vi "Problem 10.vi"() -> ()   [LabVIEW 2013, in "Problem 10.lvlib"]
uses:
  Problem 10.lvlib
  Problem 3/Problem 3.lvlib
panel:
  out "Sum of Primes <2M":u64
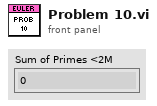
[diagram p1: front panel]
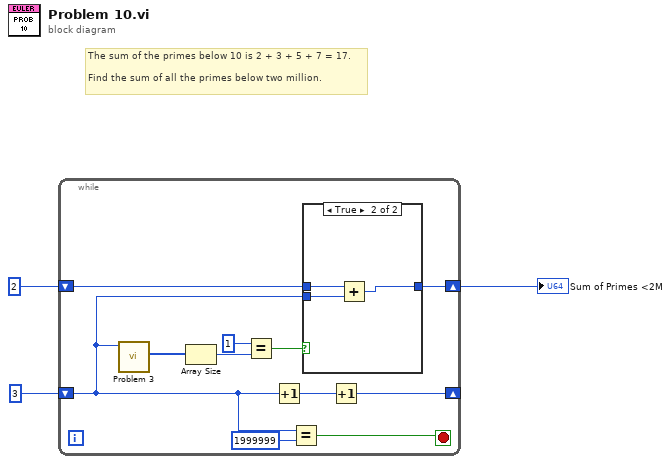
[diagram p0: block diagram]
diagram:
  # "The sum of the primes below 10 is 2 + 3 + 5 + 7 = 17.\n\nFind the sum of all the primes below two million."
  n1 = while {
    shift-right: [w7] -> _
    shift-left: u64 3 -> [w6]
    shift-right: [w9] -> w1
    shift-left: u64 2 -> [w11]
    stop <- w4 stop-if-true
    n2 = call "Problem 3.vi"("Number to Factor"=w6) -> ("List of Factors"=w14:u64[])  [unwired: 9 in, 1 out]
    n3 = Array Size(array=w14) -> (size(s)=w13:i32)
    n4 = Equal?(x=1, y=w13) -> (x = y?=w10:bool)
    n5 = Increment(x=w6) -> (x+1=w8:u64)
    n6 = Equal?(x=w6, y=u64 1999999) -> (x = y?=w4:bool)
    n7 = case shown="True" w10 {
      tunnel: w11 -> [w15 w18]
      tunnel: w6 -> [_ w17]
      tunnel: [w15 w16] -> w9
      frame False {
      }
      frame True {
        n8 = Add(x=w18, y=w17) -> (x+y=w16:u64)
      }
    }
    n9 = Increment(x=w8) -> (x+1=w7:u64)
  }
  "Sum of Primes <2M" <- w1
